vi "2100_HV Load Test w_Telegram Write_Meas iVIO.vi"(0 "Semiconductor Module Context":T3, 1 "Reg0_State":string="State00", 2 "Pins":string[](array[string])=["CLK", "SDA"], 3 "Published_Data_ID":string="HV39_", 5 "HV_Load_Steps_uA":dbl[](array[numeric])=[0.0, 5.0, 8.0, 10.0] format="%#_6p", 7 "USID":T2 max=15, 9 "Reg_Address_Data":T1 {"Address" format="%.0x"}, 11 "error in (no error)":errorcluster) -> (15 "error out":errorcluster)   [LabVIEW 2013]
uses:
  <vilib>/NI_TestStand_SemiconductorModule/NI_TestStand_Semiconductor_Module.lvlibp/PinMap/General/SemiconductorModuleContext.ctl
  Controls/USID.ctl
  Controls/Reg_Address_Data.ctl
  <vilib>/NI_TestStand_SemiconductorModule/NI_TestStand_Semiconductor_Module.lvlibp/PinMap/DC Power/PinsToNIDCPowerSessions.vi
  <vilib>/NI_TestStand_SemiconductorModule/NI_TestStand_Semiconductor_Module.lvlibp/PinMap/Deprecated/PublishDataDoubleMultiplePinsSingleInstrument.vi
  <vilib>/NI_TestStand_SemiconductorModule/NI_TestStand_Semiconductor_Module.lvlibp
panel:
  out "ReadBack Array":i32[](array[numeric])
  out "current measurements":dbl[][](array[numeric]) format="%#_6p"
  out "voltage measurements":dbl[][](array[numeric])
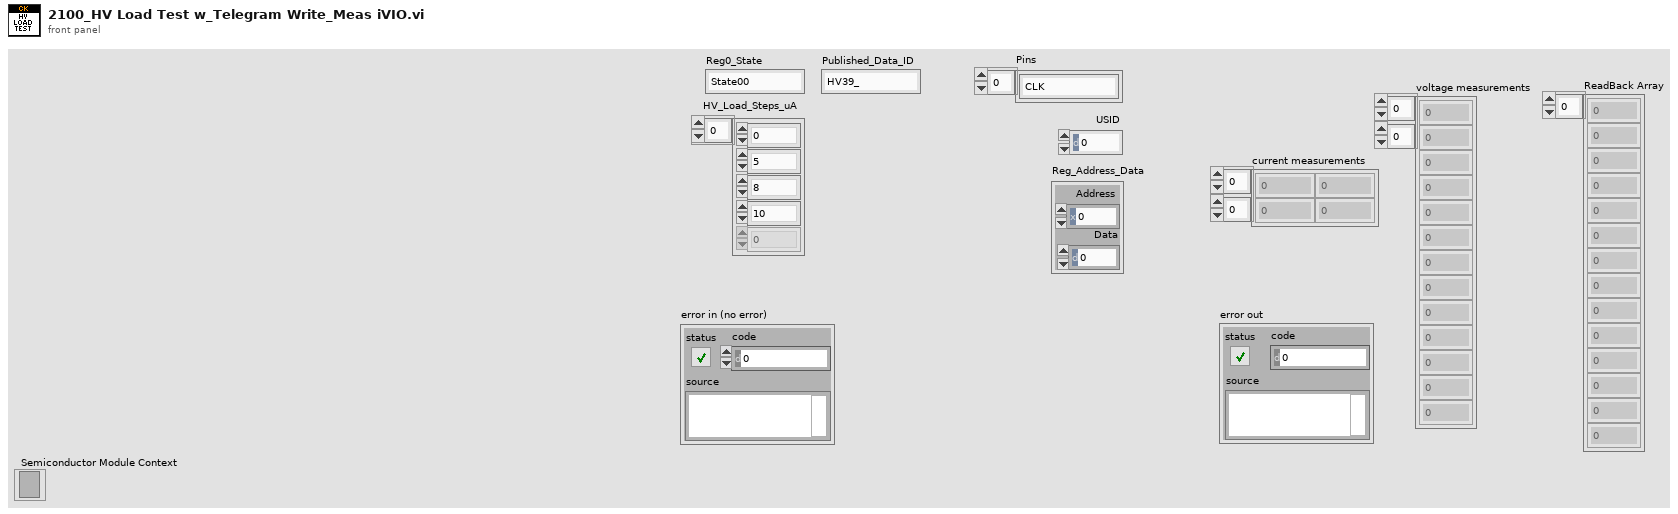
[diagram p1: front panel]
types:
  T1 = typedef "Reg_Address_Data.ctl" = cluster{"Address":u8, "Data":u8}
  T2 = typedef "USID.ctl" = u8
  T3 = typedef "NI_TestStand_Semiconductor_Module.lvlibp/SemiconductorModuleContext.ctl" = refnum<k7>
  T4 = cluster{"Slave Address":u8, "Register":u8, "Data":u8}
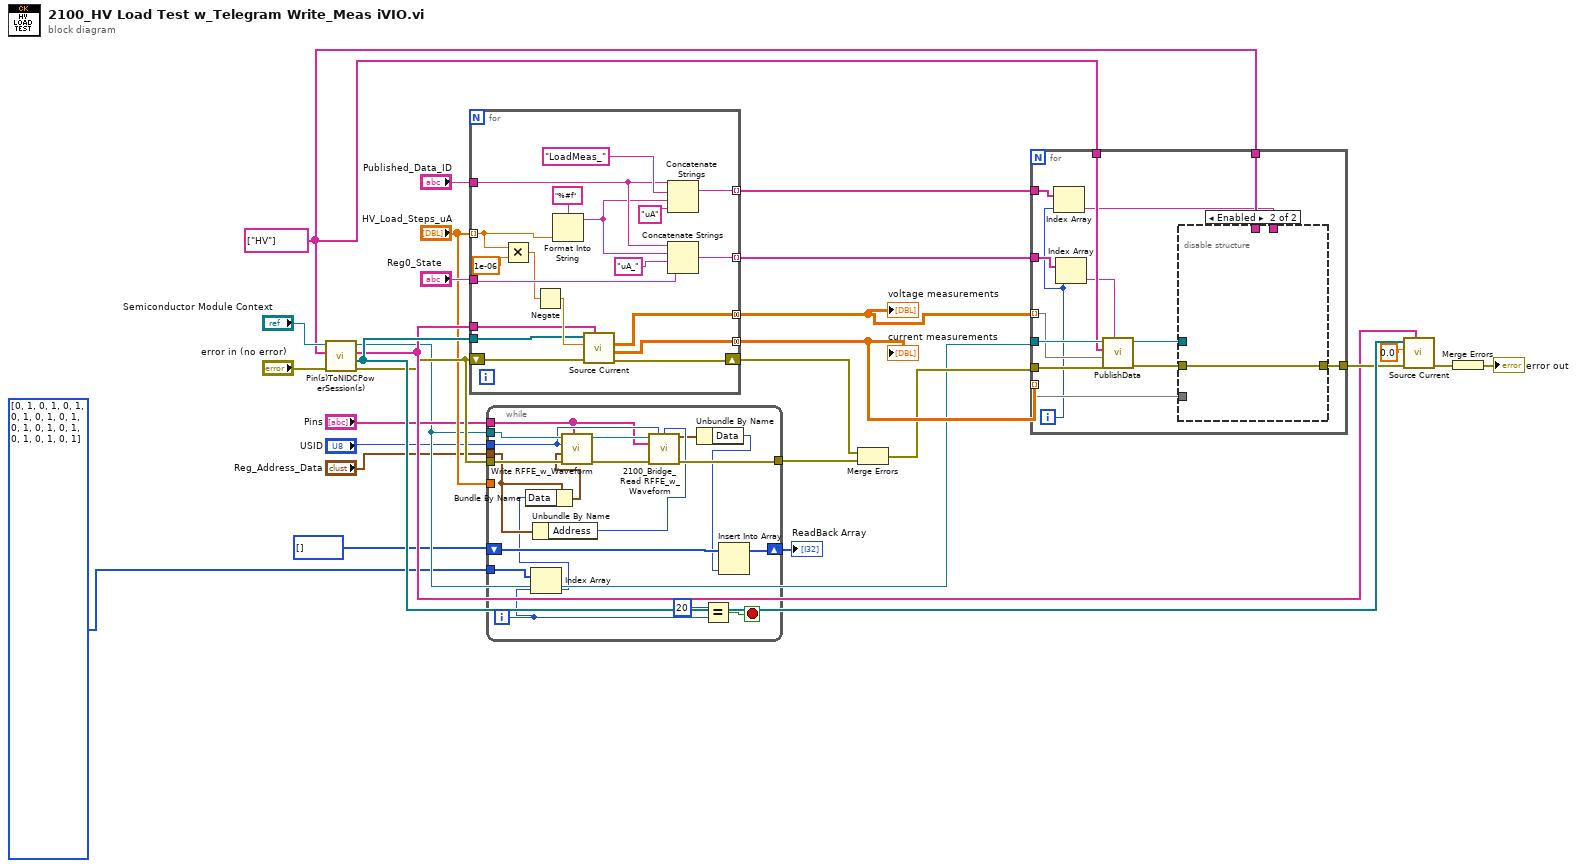
[diagram p0: block diagram]
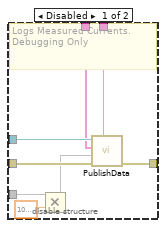
[diagram p2: hidden frame]
diagram:
  w19 = string[] ["HV"] ("Pins")
  n1 = call-poly <vilib>:"Pin(s)ToNIDCPowerSession(s).vi"("error in (no error)"="error in (no error)", "Pins"=w19, "Semiconductor Module Context"="Semiconductor Module Context") -> ("error out"=w12:errorcluster, "Instrument Sessions"=w26:refnum<k15>[], "Channel Lists"=w21:string[], "Semiconductor Module Context Out"=w6:T3)  [unwired: 4 in, 1 out]
  n2 = for {
    tunnel: w21 -> [w29]
    tunnel: "HV_Load_Steps_uA" -> [w33] mode=indexing
    tunnel: w26 -> [w30]
    shift-right: [w28] -> w9
    shift-left: w12 -> [w31]
    tunnel: "Published_Data_ID" -> [w39]
    tunnel: "Reg0_State" -> [w44]
    tunnel: [w43] -> w20 mode=concatenating
    tunnel: [w42] -> w15 mode=indexing
    tunnel: [w41] -> w18 mode=concatenating
    tunnel: [w38] -> w16 mode=indexing
    n3 = Multiply(x=w33, y=1e-06) -> (x*y=w35:dbl)
    n4 = Negate(x=w35) -> (-x=w45:dbl)
    n5 = Format Into String(format string="%#f", w33) -> (resulting string=w32:string)  [unwired: 2 in, 1 out]
    n6 = call "Source Current.vi"("Channel Lists"=w29, "error in (no error)"=w31, "current level"=w45, "Instrument Sessions In"=w30) -> ("error out"=w28:errorcluster, "current measurements"=w41:dbl[][], "voltage measurements"=w43:dbl[][])  [unwired: 4 in, 1 out]
    n7 = Concatenate Strings(w39, "LoadMeas_" ("string"), w32, "uA" ("string")) -> (w38:string)
    n8 = Concatenate Strings(w39, w32, "uA_" ("string"), w44) -> (w42:string)
  }
  "voltage measurements" <- w20
  "current measurements" <- w18
  n9 = while {
    tunnel: w12 -> [w65]
    tunnel: "HV_Load_Steps_uA" -> [_]
    tunnel: [w61] -> w10
    tunnel: "Pins" -> [w57]
    tunnel: w6 -> [w63]
    tunnel: "USID" -> [w59]
    tunnel: "Reg_Address_Data" -> [w51]
    shift-right: [w53] -> w2
    shift-left: i32[] [] -> [w55]
    tunnel: i32[] [0, 1, 0, 1, 0, 1, 0, 1, 0, 1, 0, 1, 0, 1, 0, 1, 0, 1, 0, 1, 0, 1, 0, 1] -> [w50]
    i -> [w49]
    stop <- w64 stop-if-true
    n10 = Index Array(array=w50, index=w49) -> (element=w48:i32)
    n11 = Bundle By Name(cluster=w51, "Data"=w48) -> (w47:T1)
    n12 = Unbundle By Name(w51) -> ("Address"=w58:u8)
    n13 = call "Write RFFE_w_Waveform.vi"("Pins"=w57, "error in (no error)"=w65, "Reg_Address_Data"=w47, "USID"=w59, "Semiconductor Module Context"=w63) -> ("error out"=w62:errorcluster, "Semiconductor Module Context Out"=w60:T3)  [unwired: 5 in]
    n14 = call "2100_Bridge_Read RFFE_w_Waveform.vi"("Semiconductor Module Context"=w60, "USID"=w59, "Reg Address"=w58, "Pins"=w57, "Error In"=w62) -> ("Converted Data"=w56:T4, "Error Out"=w61:errorcluster)  [unwired: 9 in]
    n15 = Unbundle By Name(w56) -> ("Data"=w54:u8)
    n16 = Equal?(x=20, y=w49) -> (x = y?=w64:bool)
    n17 = Insert Into Array(array=w55, new element=w54) -> (w53:i32[])  [unwired: 1 in]
  }
  "ReadBack Array" <- w2
  n18 = Merge Errors(w9, w10) -> (w8:errorcluster)
  n19 = for {
    tunnel: w8 -> [w79]
    tunnel: [w75] -> w22
    tunnel: w6 -> [w78]
    tunnel: w20 -> [w77] mode=indexing
    tunnel: w19 -> [w76]
    tunnel: w19 -> [w72]
    tunnel: w18 -> [w71] mode=indexing
    tunnel: w15 -> [w70]
    tunnel: w16 -> [w69]
    i -> [w66]
    n20 = Index Array(array=w69, index=w66) -> (element=w68:string)
    n21 = Index Array(array=w70, index=w66) -> (element=w67:string)
    n22 = call-poly <vilib>:"PublishData.vi"("Measurement Id"=w67, "error in (no error)"=w79, "Data In"=w77, "Pins"=w76, "Semiconductor Module Context"=w78) -> ("error out"=w74:errorcluster, "Semiconductor Module Context Out"=w73:T3)  [unwired: 5 in]
    n23 = disable-structure shown="Enabled" {
      disable-tunnel: [w87 w88] -> w75
      disable-tunnel: w74 -> [w86 w88]
      disable-tunnel: w73 -> [w85 _]
      disable-tunnel: w72 -> [w84 _]
      disable-tunnel: w71 -> [w81 _]
      disable-tunnel: w68 -> [w80 _]
      frame Disabled {
        # "Logs Measured Currents.\nDebugging Only"
        n24 = Multiply(x=w81, y=1000000.0) -> (x*y=w83:dbl[])
        n25 = call-poly <vilib>:"PublishData.vi"("Measurement Id"=w80, "error in (no error)"=w86, "Data In"=w83, "Pins"=w84, "Semiconductor Module Context"=w85) -> ("error out"=w87:errorcluster)  [unwired: 5 in, 1 out]
      }
      frame Enabled {
      }
    }
  }
  n26 = call "Source Current.vi"("Channel Lists"=w21, "error in (no error)"=w22, "current level"=0.0, "Instrument Sessions In"=w26) -> ("error out"=w14:errorcluster)  [unwired: 4 in, 3 out]
  n27 = Merge Errors(w14) -> (→"error out":errorcluster)
